vi "Keithley 24XX Custom Math Operation.vi"() -> ()   [LabVIEW 2009]
doc: "Creates a custom math operation and reads the results of the math formula applied to readings."
uses:
  <instrlib>/Keithley 24XX/Public/Data/Read (Math).vi
  <instrlib>/Keithley 24XX/Keithley 24XX.lvlib
panel:
  in  "Source Mode  (0: Voltage)":u16(ring) items=["Voltage", "Current"]
  out "Math Results":dbl[](array[numeric])
  in  "VISA resource name":refnum<visa-resource-name>
  in  "Serial Configuration":T1={"Baud Rate"=9600, "Parity"=0, "Data Bits"=8, "Stop Bits"=10, "Flow Control"=0} {"Flow Control" items=["None", "XON/XOFF", "RTS/CTS", "XON/XOFF & RTS/CTS", "DTR/DSR", "XON/XOFF & DTR/DSR"]; "Stop Bits" items=["1.0"=10, "1.5"=15, "2.0"=20]; "Data Bits" items=["7"=7, "8"=8]; "Parity" items=["None", "Odd", "Even", "Mark", "Space"]; "Baud Rate" items=["300"=300, "600"=600, "1200"=1200, "2400"=2400, "4800"=4800, "9600"=9600, "19200"=19200]}
  in  "Sample Count (5)":i32=5
  in  "Timeout (10000 ms)":i32=10000 format="%#.6g"
  in  "Compliance  Level (0.1)":dbl=0.1
  in  "Output Level (0)":dbl
  # "(c) 2006 National Instruments.  ALL RIGHTS RESERVED."
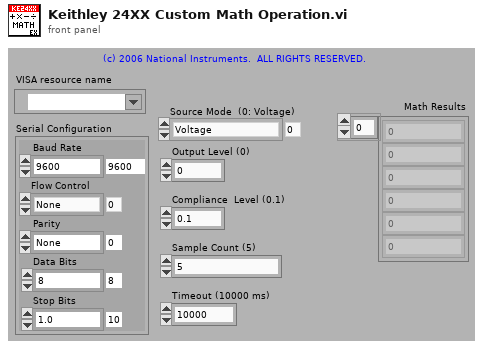
[diagram p1: front panel]
types:
  T1 = cluster{"Baud Rate":u32, "Parity":u16, "Data Bits":u16, "Stop Bits":u16, "Flow Control":u16}
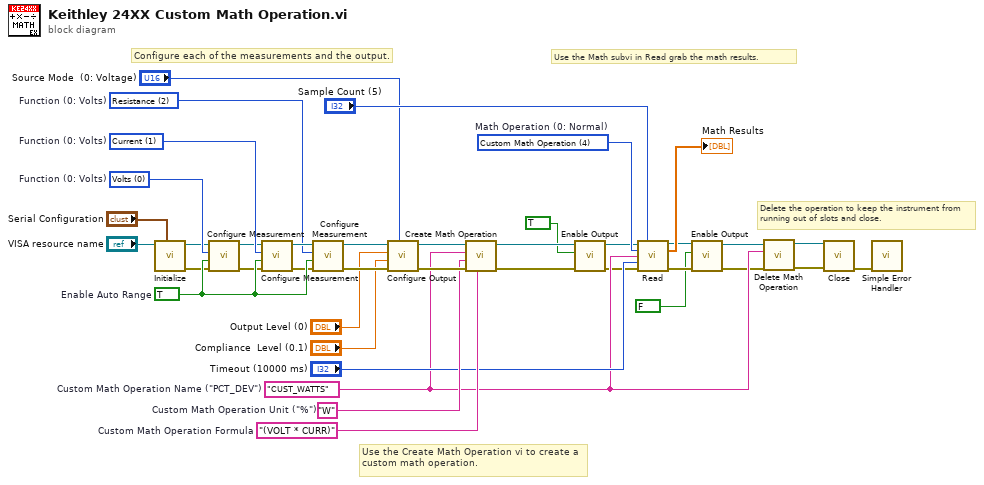
[diagram p0: block diagram]
diagram:
  w19 = u16 4 items=["Power", "Offset Compensated Ohms", "Resistor Voltage Coefficient", "Varistor Alpha", "Custom Math Operation"]  # Math Operation (0: Normal)
  w20 = "(VOLT * CURR)"  # Custom Math Operation Formula
  w21 = "W"  # Custom Math Operation Unit ("%")
  w15 = "CUST_WATTS"  # Custom Math Operation Name ("PCT_DEV")
  w25 = u16 2 items=["Volts", "Current", "Resistance"]  # Function (0: Volts)
  w37 = u16 1 items=["Volts", "Current", "Resistance"]  # Function (0: Volts)
  w36 = u16 0 items=["Volts", "Current", "Resistance"]  # Function (0: Volts)
  w35 = TRUE  # Enable Auto Range
  # "Delete the operation to keep the instrument from running out of slots and close."
  # "Use the Math subvi in Read grab the math results."
  # "Use the Create Math Operation vi to create a custom math operation."
  # "Configure each of the measurements and the output."
  n1 = call <instrlib>:"Initialize.vi"("Serial Configuration"="Serial Configuration", "VISA resource name"="VISA resource name") -> ("error out"=w29:errorcluster, "VISA resource name out"=w28:refnum<visa-resource-name>)  [unwired: 8 in]
  n2 = call <instrlib>:"Configure Measurement.vi"("error in (no error)"=w29, "Enable Auto Range (T:Enable)"=w35, "Function (0: Volts)"=w36, "VISA resource name"=w28) -> ("error out"=w31:errorcluster, "VISA resource name out"=w32:refnum<visa-resource-name>)  [unwired: 6 in]
  n3 = call <instrlib>:"Configure Measurement.vi"("error in (no error)"=w31, "Enable Auto Range (T:Enable)"=w35, "Function (0: Volts)"=w37, "VISA resource name"=w32) -> ("error out"=w34:errorcluster, "VISA resource name out"=w33:refnum<visa-resource-name>)  [unwired: 6 in]
  n4 = call <instrlib>:"Configure Measurement.vi"("error in (no error)"=w34, "Enable Auto Range (T:Enable)"=w35, "Function (0: Volts)"=w25, "VISA resource name"=w33) -> ("error out"=w39:errorcluster, "VISA resource name out"=w38:refnum<visa-resource-name>)  [unwired: 6 in]
  n5 = call <instrlib>:"Configure Output.vi"("Source Mode  (0: Voltage)"="Source Mode  (0: Voltage)", "error in (no error)"=w39, "Compliance  Level (0.1)"="Compliance  Level (0.1)", "Output Level (0)"="Output Level (0)", "VISA resource name"=w38) -> ("error out"=w23:errorcluster, "VISA resource name out"=w22:refnum<visa-resource-name>)  [unwired: 5 in]
  n6 = call <instrlib>:"Create Math Operation.vi"("Custom Math Operation Formula (\"(((RES - 10e3)/10e3)*100)\")"=w20, "error in (no error)"=w23, "Custom Math Operation Unit (\"%\")"=w21, "Custom Math Operation Name (\"PCT_DEV\")"=w15, "VISA resource name"=w22) -> ("error out"=w10:errorcluster, "VISA resource name out"=w11:refnum<visa-resource-name>)  [unwired: 5 in]
  n7 = call <instrlib>:"Enable Output.vi"("error in (no error)"=w10, "Enable Output (T: Enable)"=TRUE, "VISA resource name"=w11) -> ("error out"=w9:errorcluster, "VISA resource name out"=w8:refnum<visa-resource-name>)  [unwired: 7 in]
  n8 = call-poly <instrlib>:"Read.vi"("VISA resource name"=w8, "Sample Count (1)"="Sample Count (5)", "Math Operation (0: Power)"=w19, "Custom Math Operation Name (\"Custom\")"=w15, "Timeout (10000 ms)"="Timeout (10000 ms)", "error in (no error)"=w9) -> ("VISA resource name out"=w6:refnum<visa-resource-name>, "Math Results"=→"Math Results":dbl[], "error out"=w7:errorcluster)  [unwired: 7 in]
  n9 = call <instrlib>:"Enable Output.vi"("error in (no error)"=w7, "Enable Output (T: Enable)"=FALSE, "VISA resource name"=w6) -> ("error out"=w4:errorcluster, "VISA resource name out"=w5:refnum<visa-resource-name>)  [unwired: 7 in]
  n10 = call <instrlib>:"Delete Math Operation.vi"("error in (no error)"=w4, "Custom Math Operation Name (\"PCT_DEV\")"=w15, "VISA resource name"=w5) -> ("error out"=w17:errorcluster, "VISA resource name out"=w16:refnum<visa-resource-name>)  [unwired: 7 in]
  n11 = call <instrlib>:"Close.vi"("error in (no error)"=w17, "VISA resource name"=w16) -> ("error out"=w26:errorcluster)  [unwired: 9 in]
  n12 = call <vilib>:"Simple Error Handler.vi"("error in (no error)"=w26) -> ()  [unwired: 4 in, 5 out]
